vi "Create_Trajectory_Make_Trajectory.vi"(6 "TRAJECTORY_CONFIG":T1 {"End Velocity" format="%20.4f"; "StartVelocity" format="%20.4f"; "Max Acceleration" format="%20.4f"; "MaxVelocity" format="%20.4f"}, 9 "Spline Type":enum32{"Radio Selection 1", "Radio Selection 2"}(ring), 10 "WayPoints":T2[](array[typedef]) {"WEIGHT" format="%13.3f"; "ANGLE" format="%13.3f"; "Y" format="%13.3f"; "X" format="%13.3f"}, 11 "UseWeights":bool) -> (0 "error out":errorcluster, 2 "Is Cubic":bool, 3 "TRAJECTORY":T3 {"States"."POSE"."ROTATION"."SIN" format="%13.4f"; "States"."POSE"."ROTATION"."COS" format="%13.4f"; "States"."POSE"."ROTATION"."VALUE" format="%13.4f"; "States"."POSE"."TRANSLATION"."Y" format="%14.3f"; "States"."POSE"."TRANSLATION"."X" format="%14.3f"; "TotalTImeSecs" format="%20.3f"})   [LabVIEW 2019]
uses:
  <vilib>/Rock Robotics/WPI/ThirdParty/JAS_Junk/TrajLib/TypeDef/TRAJECTORY.ctl
  <vilib>/Rock Robotics/WPI/ThirdParty/JAS_Junk/TrajLib/TypeDef/TRAJ_STATE.ctl
  <vilib>/Rock Robotics/WPI/ThirdParty/JAS_Junk/TrajLib/TypeDef/POSE2D.ctl
  <vilib>/Rock Robotics/WPI/ThirdParty/JAS_Junk/TrajLib/TypeDef/TRANSLATION2D.ctl
  <vilib>/Rock Robotics/WPI/ThirdParty/JAS_Junk/TrajLib/TypeDef/ROTATION2D.ctl
  <vilib>/Rock Robotics/WPI/ThirdParty/JAS_Junk/TrajLib/TypeDef/DISPLAY_WEIGHTED_WAYPOINT.ctl
  <vilib>/Rock Robotics/WPI/ThirdParty/JAS_Junk/TrajLib/TypeDef/TRAJ_CONFIG.ctl
  <vilib>/Rock Robotics/WPI/ThirdParty/JAS_Junk/TrajLib/Translation2d_Create.vi
  <vilib>/Rock Robotics/WPI/ThirdParty/JAS_Junk/TrajLib/Rotation2d_CreateAngle.vi
  <vilib>/Rock Robotics/WPI/ThirdParty/JAS_Junk/TrajLib/Trajectory_Library.lvlib
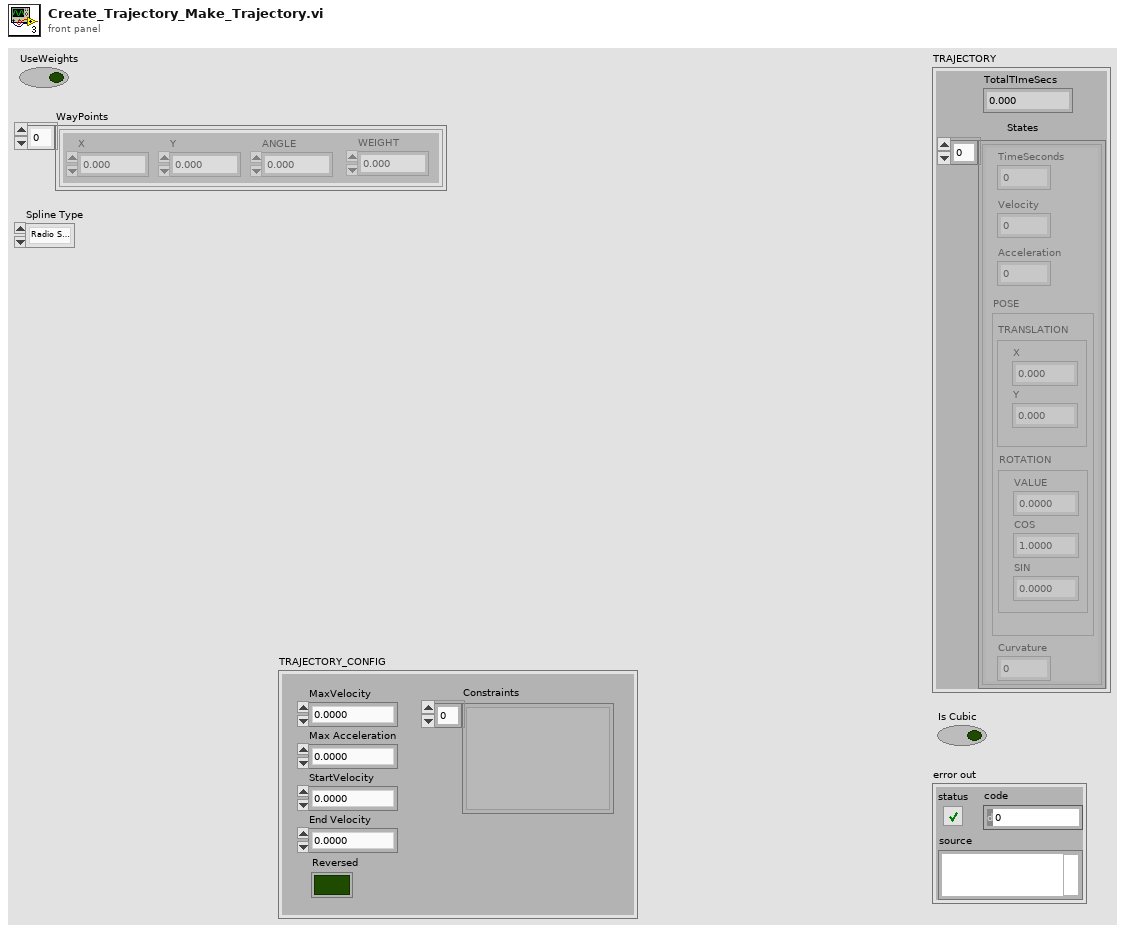
[diagram p1: front panel]
types:
  T1 = typedef "Trajectory_Library.lvlib/TRAJ_CONFIG.ctl" = cluster{"MaxVelocity":dbl, "Max Acceleration":dbl, "StartVelocity":dbl, "End Velocity":dbl, "Reversed":bool, "Constraints":variant[]}
  T2 = typedef "Trajectory_Library.lvlib/DISPLAY_WEIGHTED_WAYPOINT.ctl" = cluster{"X":dbl, "Y":dbl, "ANGLE":dbl, "WEIGHT":dbl}
  T3 = typedef "Trajectory_Library.lvlib/TRAJECTORY.ctl" = cluster{"TotalTImeSecs":dbl, "States":T4[]}
  T4 = typedef "Trajectory_Library.lvlib/TRAJ_STATE.ctl" = cluster{"TimeSeconds":dbl, "Velocity":dbl, "Acceleration":dbl, "POSE":T5, "Curvature":dbl}
  T5 = typedef "Trajectory_Library.lvlib/POSE2D.ctl" = cluster{"TRANSLATION":T6, "ROTATION":T7}
  T6 = typedef "Trajectory_Library.lvlib/TRANSLATION2D.ctl" = cluster{"X":dbl, "Y":dbl}
  T7 = typedef "Trajectory_Library.lvlib/ROTATION2D.ctl" = cluster{"VALUE":dbl, "COS":dbl, "SIN":dbl}
  T8 = typedef "Trajectory_Library.lvlib/WEIGHTED_WAYPOINT.ctl" = cluster{"TRANSLATION":T6, "ROTATION":T7, "SCALAR":dbl}
  T9 = typedef "Trajectory_Library.lvlib/SPLINE_CTRL_VECTOR.ctl" = cluster{"Xs":dbl[], "Ys":dbl[]}
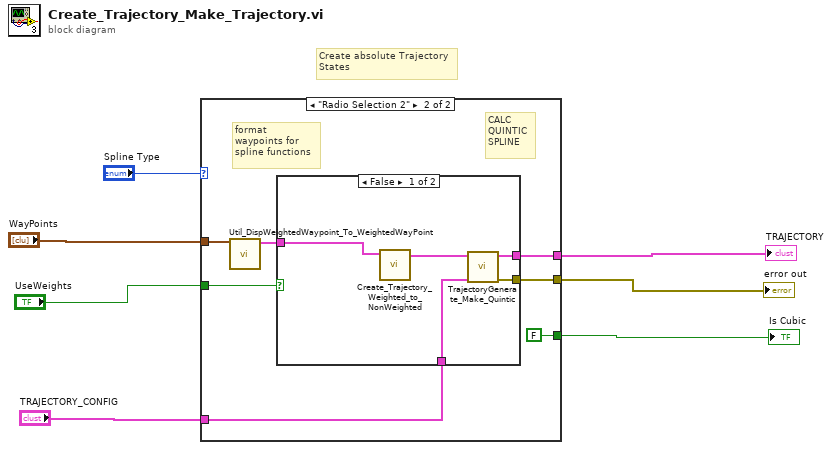
[diagram p0: block diagram]
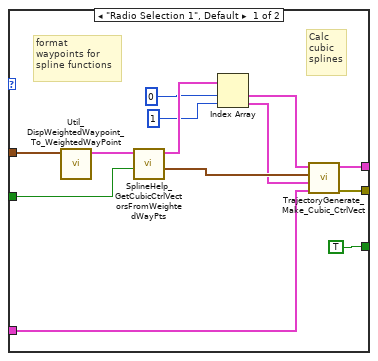
[diagram p2: hidden frame]
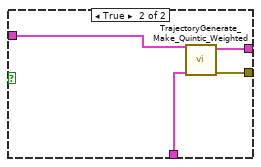
[diagram p3: hidden frame]
diagram:
  # "Create absolute Trajectory\nStates"
  n1 = case shown="\"Radio Selection 2\"" "Spline Type" {
    tunnel: [w19 w23] -> w1
    tunnel: "TRAJECTORY_CONFIG" -> [w18 w22]
    tunnel: [w20 w24] -> w7
    tunnel: [TRUE FALSE] -> w3
    tunnel: "WayPoints" -> [w16 w26]
    tunnel: "UseWeights" -> [w10 w21]
    frame "Radio Selection 1", Default {
      # "format\nwaypoints for\nspline functions"
      # "Calc\ncubic\nsplines"
      n2 = call <vilib>:"Util_DispWeightedWaypoint_To_WeightedWayPoint.vi"("DisplayWeightedWayPoints"=w16) -> ("WeightedWayPoints"=w15:T8[])  [unwired: 10 in]
      n3 = call <vilib>:"SplineHelp_GetCubicCtrlVectorsFromWeightedWayPts.vi"("Use Weights"=w10, "WeightedWayPoints"=w15) -> ("Interior WAYPOINTS"=w14:T6[], "SplineControlVectors"=w13:T9[])  [unwired: 8 in]
      n4 = Index Array(array=w13, index #1=0 ("index"), index #2=1 ("index")) -> (element #1=w12:T9, element #2=w11:T9)
      n5 = call <vilib>:"TrajectoryGenerate_Make_Cubic_CtrlVect.vi"("traj_config"=w18, "end-Spline_Ctrl_Vector"=w11, "Interior WAYPOINTS"=w14, "initial-Spline_Ctrl_Vector"=w12) -> ("error out"=w19:errorcluster, "TRAJECTORY"=w20:T3)  [unwired: 6 in]
    }
    frame "Radio Selection 2" {
      # "format\nwaypoints for\nspline functions"
      # "CALC\nQUINTIC\nSPLINE"
      n6 = call <vilib>:"Util_DispWeightedWaypoint_To_WeightedWayPoint.vi"("DisplayWeightedWayPoints"=w26) -> ("WeightedWayPoints"=w25:T8[])  [unwired: 10 in]
      n7 = case shown="False" w21 {
        tunnel: [w32 w36] -> w24
        tunnel: [w31 w35] -> w23
        tunnel: w25 -> [w28 w34]
        tunnel: w22 -> [w29 w33]
        frame False {
          n8 = call "Create_Trajectory_Weighted_to_NonWeighted.vi"("WeightedWayPoints"=w28) -> ("WayPoints"=w30:T5[])  [unwired: 10 in]
          n9 = call <vilib>:"TrajectoryGenerate_Make_Quintic.vi"("traj_config"=w29, "waypointPOSE"=w30) -> ("error out"=w31:errorcluster, "TRAJECTORY"=w32:T3)  [unwired: 8 in]
        }
        frame True {
          n10 = call <vilib>:"TrajectoryGenerate_Make_Quintic_Weighted.vi"("traj_config"=w33, "WeightedWaypointPOSE"=w34) -> ("error out"=w35:errorcluster, "TRAJECTORY"=w36:T3)  [unwired: 8 in]
        }
      }
    }
  }
  "TRAJECTORY" <- w7
  "Is Cubic" <- w3
  "error out" <- w1
